vi "Angle Corrected Coordinates.vi"(4 "Outer iteration":dbl, 5 "Inner iteration":dbl, 6 "Corrected angle":dbl, 7 "Pitch (um)":dbl) -> (1 "Correction angle (deg)":dbl format="%#.9g", 2 "y position":dbl, 3 "x position":dbl)   [LabVIEW 2022 SP3]
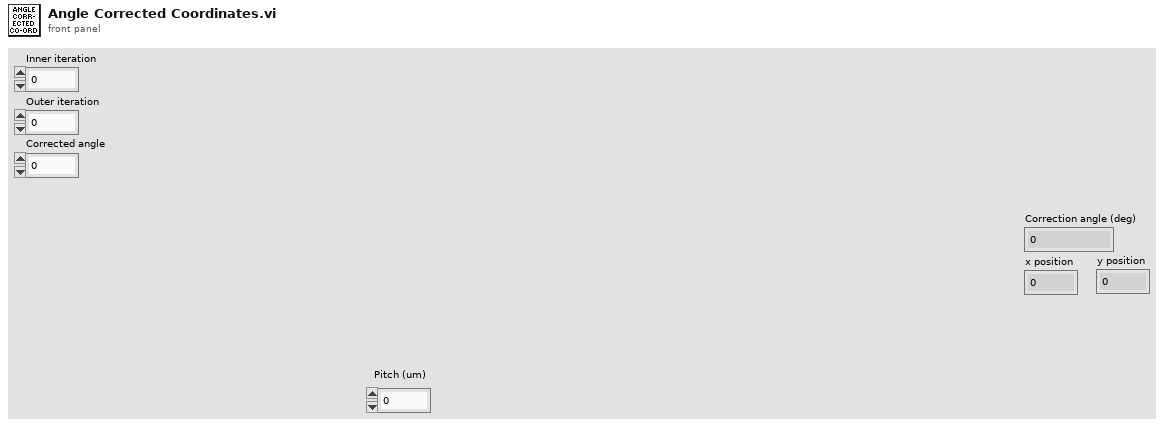
[diagram p1: front panel]
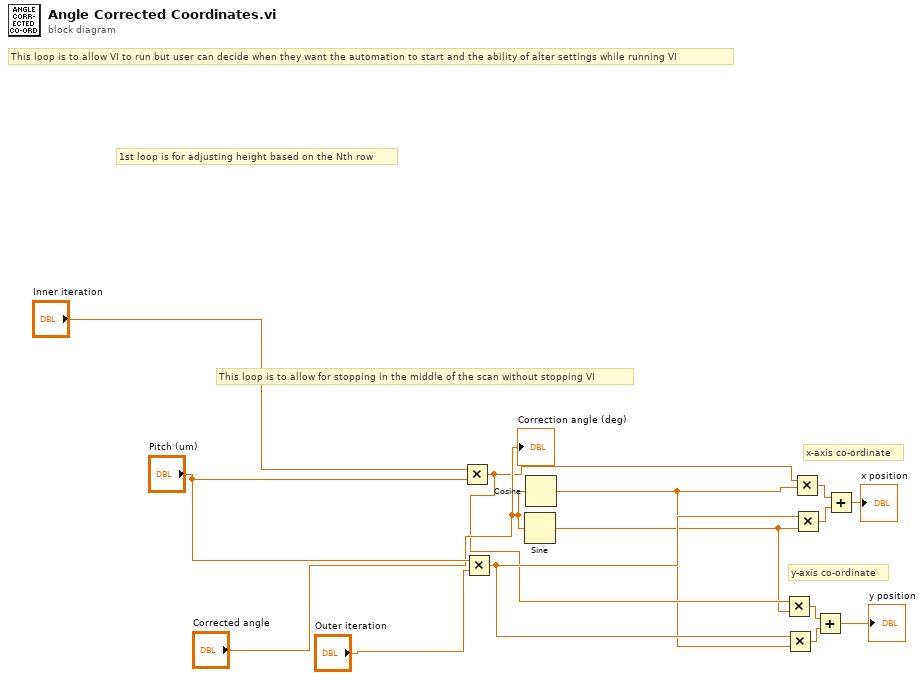
[diagram p0: block diagram]
diagram:
  # "This loop is to allow for stopping in the middle of the scan without stopping VI"
  # "y-axis co-ordinate"
  # "x-axis co-ordinate"
  # "1st loop is for adjusting height based on the Nth row"
  # "This loop is to allow VI to run but user can decide when they want the automation to start and the ability of alter settings while running VI"
  n1 = Multiply(x="Inner iteration", y="Pitch (um)") -> (x*y=w3:dbl)
  n2 = Multiply(x="Pitch (um)", y="Outer iteration") -> (x*y=w10:dbl)
  n3 = Sine(x="Corrected angle") -> (sin(x)=w2:dbl)
  n4 = Cosine(x="Corrected angle") -> (cos(x)=w1:dbl)
  n5 = Multiply(x=w3, y=w2) -> (x*y=w9:dbl)
  n6 = Multiply(x=w10, y=w1) -> (x*y=w8:dbl)
  n7 = Multiply(x=w3, y=w1) -> (x*y=w13:dbl)
  n8 = Multiply(x=w10, y=w2) -> (x*y=w12:dbl)
  n9 = Add(x=w9, y=w8) -> (x+y=→"y position":dbl)
  n10 = Add(x=w13, y=w12) -> (x+y=→"x position":dbl)
  "Correction angle (deg)" <- "Corrected angle"
